vi "BB_Image_Process.vi"(9 "Color Controls":T3={"Hue"={107.81818389892578, 139.81818389892578}, "Sat"={176.07142857142858, 255.0}, "Val"={40.53571428571429, 255.0}} {"Hue" scale=0.0..255.0 scale format="%#_3g"}, 10 "Mask":T2, 11 "Input Image":T2) -> (1 "Results":T4 {"Score" format="%#_3g"; "Pixels"."Rectangle"."Numeric 5" format="%#_3g"; "Pixels"."Rectangle"."Numeric 3" format="%#_3g"; "Pixels"."Rectangle"."Numeric 2" format="%#_3g"; "Pixels"."Rectangle"."Numeric" format="%#_3g"; "Normalized"."Rectangle"."Numeric 5" format="%#_2g"; "Normalized"."Rectangle"."Numeric 3" format="%#_2g"; "Normalized"."Rectangle"."Numeric 2" format="%#_2g"; "Normalized"."Rectangle"."Numeric" format="%#_2g"; "Normalized"."Center"."?" format="%#_3g"; "Normalized"."Center"."?" format="%#_3g"; "Distance (ft)" format="%#_3g"}, 2 "Mask":T2(plugin-control), 3 "Original Image":T2(plugin-control))   [LabVIEW 2016]
uses:
  Vision Support Code/Camera Types.ctl
  <vilib>/vision/Image Controls.llb/IMAQ Image.ctl
  <vilib>/vision/NI_Vision_Development_Module.lvlib
panel:
  in  "Dilate":bool=TRUE
  in  "Operation 2":T1(ring)=enum."Erode"
  in  "Operation":T1(ring)=enum."Dilate"
  in  "Number of iterations (1) 2":i32=1
  in  "Number of iterations (1)":i32=1
  out "Qualified Particles":i32
  in  "Annotate":bool=TRUE
  in  "Camera Type":T5=enum."MS HD3000 square"
  in  "Score Cutoff %":dbl=70.0
  in  "Particles":dbl=5.0
  in  "Color Mode":u16(ring)=3 items=["RGB", "HSL", "HSV", "HSI"]
  in  "Use Calibration":bool=TRUE
  in  "Line Border":cluster{"Top":dbl, "Bottom":dbl}={"Top"=6.0, "Bottom"=1.0}
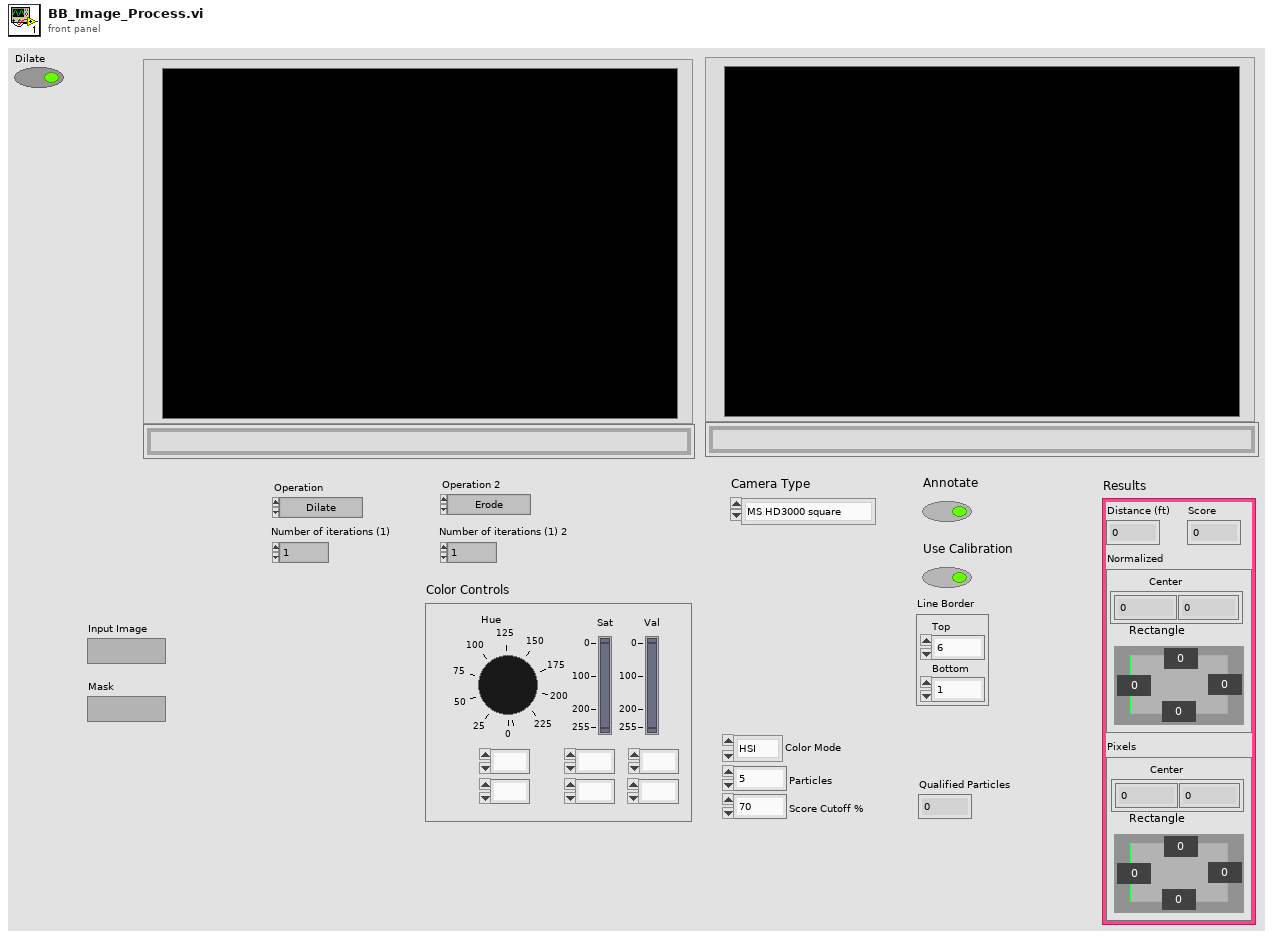
[diagram p1: front panel]
types:
  T1 = enum32{"AutoM", "Close", "Dilate", "Erode", "Gradient", "Gradient out", "Gradient in", "Hit miss", "Open", "PClose", "POpen", "Thick", "Thin"}
  T2 = typedef "IMAQ Image.ctl" = refnum<image>
  T3 = cluster{"Hue":cluster{dbl, dbl}, "Sat":cluster{dbl, dbl}, "Val":cluster{dbl, dbl}}
  T4 = cluster{"Distance (ft)":dbl, "Score":dbl, "Normalized":cluster{"Center":cluster{dbl, dbl}, "Rectangle":cluster{"Numeric":dbl, "Numeric 2":dbl, "Numeric 3":dbl, "Numeric 5":dbl}}, "Pixels":cluster{"Center":cluster{dbl, dbl}, "Rectangle":cluster{"Numeric":dbl, "Numeric 2":dbl, "Numeric 3":dbl, "Numeric 5":dbl}}}
  T5 = typedef "Camera Types.ctl" = enum16{"206", "1011", "1013", "MS HD3000 square", "MS HD3000 640x480"}
  T6 = typedef "Image Type" = u32
  T7 = typedef "Particle Parameters" = i32
  T8 = cluster{"Left":dbl, "Top":dbl, "Right":dbl, "Bottom":dbl}
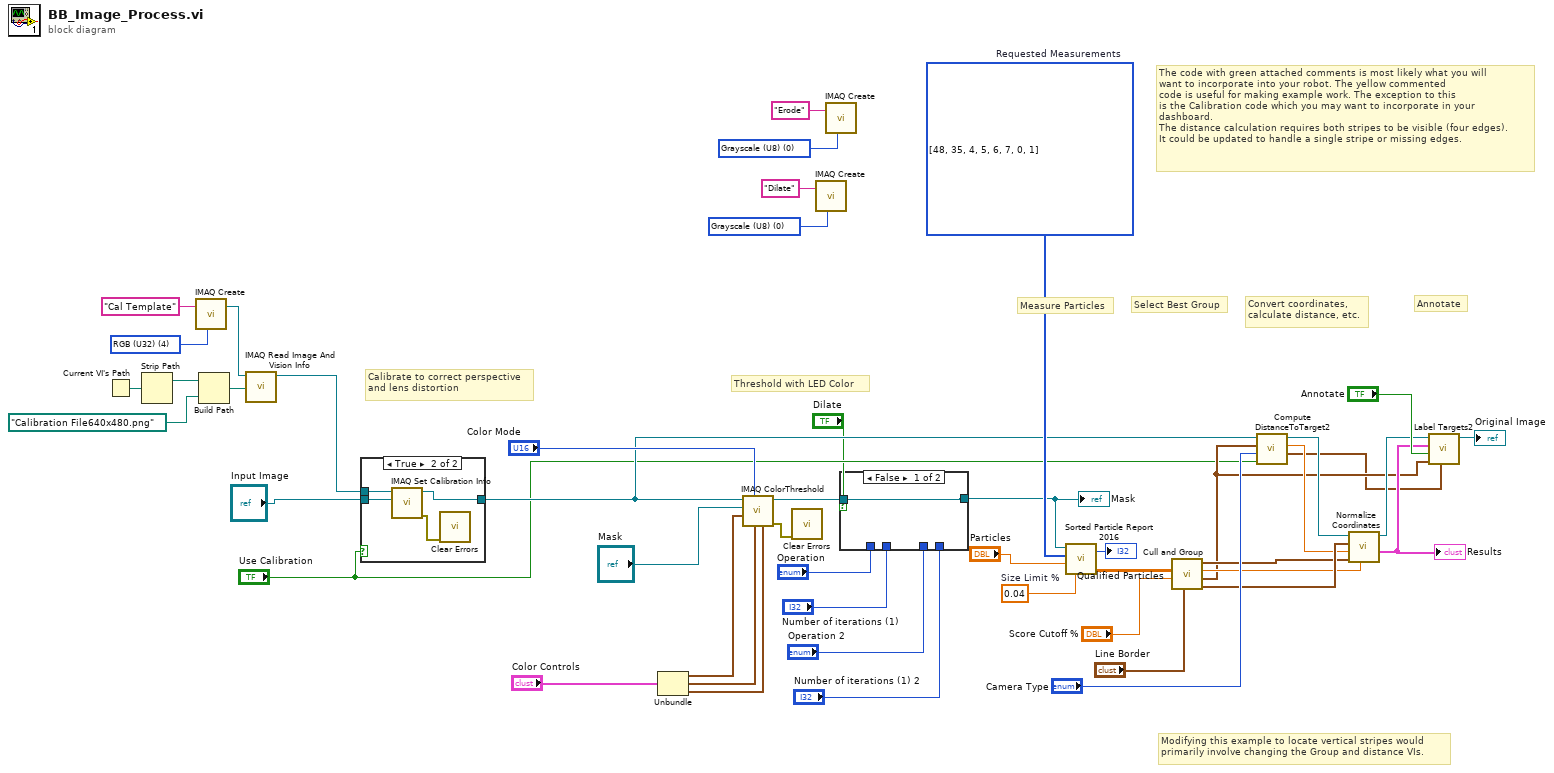
[diagram p0: block diagram]
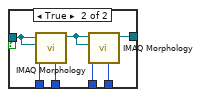
[diagram p2: hidden frame]
diagram:
  w6 = T6 0 items=["Grayscale (U8)", "Grayscale (I16)", "Grayscale (SGL)", "Complex (CSG)", "RGB (U32)", "HSL (U32)", "RGB (U64)", "Grayscale (U16)"] ("Image Type")
  w8 = T6 0 items=["Grayscale (U8)", "Grayscale (I16)", "Grayscale (SGL)", "Complex (CSG)", "RGB (U32)", "HSL (U32)", "RGB (U64)", "Grayscale (U16)"] ("Image Type")
  w35 = 0.04  # Size Limit %
  w47 = T6 4 items=["Grayscale (U8)", "Grayscale (I16)", "Grayscale (SGL)", "Complex (CSG)", "RGB (U32)", "HSL (U32)", "RGB (U64)", "Grayscale (U16)"] ("Image Type")
  w48 = T7[] [48, 35, 4, 5, 6, 7, 0, 1] items=["Center of Mass X", "Center of Mass Y", "First Pixel X", "First Pixel Y", "Bounding Rect Left", "Bounding Rect Top", "Bounding Rect Right", "Bounding Rect Bottom", "Max Feret Diameter Start X", "Max Feret Diameter Start Y", "Max Feret Diameter End X", "Max Feret Diameter End Y", "Max Horiz. Segment Length Left", "Max Horiz. Segment Length Right", "Max Horiz. Segment Length Row", "-", "Bounding Rect Width", "Bounding Rect Height", "Bounding Rect Diagonal", "Perimeter", "Convex Hull Perimeter", "Holes' Perimeter", "Max Feret Diameter", "Equivalent Ellipse Major Axis", "Equivalent Ellipse Minor Axis", "Equivalent Ellipse Minor Axis (Feret)", "Equivalent Rect Long Side", "Equivalent Rect Short Side", "Equivalent Rect Diagonal", "Equivalent Rect Short Side (Feret)", "Average Horiz. Segment Length", "Average Vert. Segment Length", "Hydraulic Radius", "Waddel Disk Diameter", "-", "Area", "Holes' Area", "Particle & Holes' Area", "Convex Hull Area", "Image Area", "-", "Number of Holes", "Number of Horiz. Segments", "Number of Vert. Segments", "-", "Orientation", "Max Feret Diameter Orientation", "-", "% Area/Image Area", "% Area/(Particle & Holes' Area)", "Ratio of Equivalent Ellipse Axes", "Ratio of Equivalent Rect Sides", "-", "Elongation Factor", "Compactness Factor", "Heywood Circularity Factor", "Type Factor", "-", "Sum X", "Sum Y", "Sum XX", "Sum XY", "Sum YY", "Sum XXX", "Sum XXY", "Sum XYY", "Sum YYY", "-", "Moment of Inertia XX", "Moment of Inertia XY", "Moment of Inertia YY", "Moment of Inertia XXX", "Moment of Inertia XXY", "Moment of Inertia XYY", "Moment of Inertia YYY", "Norm. Moment of Inertia XX", "Norm. Moment of Inertia XY", "Norm. Moment of Inertia YY", "Norm. Moment of Inertia XXX", "Norm. Moment of Inertia XXY", "Norm. Moment of Inertia XYY", "Norm. Moment of Inertia YYY", "Hu Moment 1", "Hu Moment 2", "Hu Moment 3", "Hu Moment 4", "Hu Moment 5", "Hu Moment 6", "Hu Moment 7"]  # Requested Measurements
  # "Calibrate to correct perspective\nand lens distortion"
  # "Measure Particles"
  # "Convert coordinates,\ncalculate distance, etc."
  # "Annotate"
  # "Select Best Group"
  # "Threshold with LED Color"
  # "Modifying this example to locate vertical stripes would\nprimarily involve changing the Group and distance VIs."
  # "The code with green attached comments is most likely what you will\nwant to incorporate into your robot. The yellow commented\ncode is useful for making example work. The exception to this\nis the Calibration code which you may want to incorporate in your\ndashboard.\nThe distance calculation requires both stripes to be visible (four edges).\nIt could be updated to handle a single stripe or missing edges."
  n1 = Current VI's Path() -> (path=w43:path)
  n2 = Strip Path(path=w43) -> (stripped path=w40:path)  [unwired: 1 out]
  n3 = call "IMAQ Create"("Image Name"="Cal Template", "Image Type"=w47) -> ("New Image"=w45:T2)  [unwired: 2 in, 2 out]
  n4 = Build Path(base path=w40, name or relative path=path "Calibration File640x480.png" ("Folder Location")) -> (appended path=w42:path)
  n5 = call "IMAQ Read Image And Vision Info"("File Path"=w42, "Image"=w45) -> ("Image Out"=w44:T2)  [unwired: 7 in, 2 out]
  n6 = case shown="True" "Use Calibration" {
    tunnel: [w49 w53] -> w16
    tunnel: "Input Image" -> [w49 w50]
    tunnel: w44 -> [_ w52]
    frame False {
    }
    frame True {
      n7 = call "IMAQ Set Calibration Info"("Image Dst"=w50, "Image Src"=w52) -> ("error out"=w51:errorcluster, "Calibrated Image"=w53:T2)  [unwired: 8 in]
      n8 = call <vilib>:"Clear Errors.vi"("error in (no error)"=w51) -> ()  [unwired: 5 in, 2 out]
    }
  }
  n9 = Unbundle("Color Controls") -> ("Hue"=w39:cluster{dbl, dbl}, "Sat"=w38:cluster{dbl, dbl}, "Val"=w37:cluster{dbl, dbl})
  n10 = call "IMAQ ColorThreshold"("Blue or Luma or Val or Inten Range"=w37, "Green or Sat Range"=w38, "Color Mode"="Color Mode", "Red or Hue Range"=w39, "Image Dst"="Mask", "Image Src"=w16) -> ("error out"=w32:errorcluster, "Image Dst Out"=w2:T2)  [unwired: 4 in]
  n11 = call <vilib>:"Clear Errors.vi"("error in (no error)"=w32) -> ()  [unwired: 5 in, 2 out]
  n12 = call "IMAQ Create"("Image Name"="Dilate", "Image Type"=w8) -> ()  [unwired: 2 in, 3 out]
  n13 = call "IMAQ Create"("Image Name"="Erode", "Image Type"=w6) -> ()  [unwired: 2 in, 3 out]
  n14 = case shown="False" "Dilate" {
    tunnel: "Number of iterations (1)" -> [_ w61]
    tunnel: [w54 w60] -> w10
    tunnel: "Number of iterations (1) 2" -> [_ w59]
    tunnel: "Operation" -> [_ w58]
    tunnel: "Operation 2" -> [_ w57]
    tunnel: w2 -> [w54 w56]
    frame False {
    }
    frame True {
      n15 = call "IMAQ Morphology"("Number of iterations (1)"=w61, "Operation"=w58, "Image Dst"=w56, "Image Src"=w56) -> ("Image Dst Out"=w55:T2)  [unwired: 6 in, 1 out]
      n16 = call "IMAQ Morphology"("Number of iterations (1)"=w59, "Operation"=w57, "Image Dst"=w55, "Image Src"=w55) -> ("Image Dst Out"=w60:T2)  [unwired: 6 in, 1 out]
    }
  }
  "Mask" <- w10
  n17 = call "Sorted Particle Report 2016.vi"("Min Area Size %"=w35, "Particle Count Limit"="Particles", "Pixel Measurements"=w48, "Image in"=w10) -> ("Sorted Data"=w30:dbl[][], "Particles"=→"Qualified Particles":i32)
  n18 = call "Cull and Group.vi"("Line Border"="Line Border", "Score Cutoff"="Score Cutoff %", "Sorted Data"=w30) -> ("Rect"=w27:T8, "Line"=w18:T8, "Score"=w21:dbl, "Center"=w23:cluster{"X":dbl, "Y":dbl})  [unwired: 5 in]
  n19 = call "Compute DistanceToTarget2.vi"("Calibrated"="Use Calibration", "Camera Type"="Camera Type", "Line"=w18, "Image Src"=w16) -> ("Edges"=w17:cluster{"X":sgl, "Y":sgl}[], "Distance (ft)"=w26:dbl, "Image Dst Out"=w25:T2)  [unwired: 5 in]
  n20 = call "Normalize Coordinates.vi"("Score"=w21, "Center"=w23, "Distance"=w26, "Bounding box"=w27, "Image in"=w25) -> ("Results"=w22:T4, "Image out"=w24:T2)  [unwired: 5 in]
  "Results" <- w22
  n21 = call "Label Targets2.vi"("Edges"=w17, "Line"=w18, "Annotate"="Annotate", "Results"=w22, "Image in"=w24) -> ("Image out"=→"Original Image":T2)  [unwired: 6 in]
